vi "Write_From_Dash_Values_To_NT_Ready_Arrays.vi"(0 "Pages":refnum<vi>[](array[refnum])) -> (1 "Names":string[](array[string]), 2 "Values":string[](array[string]))   [LabVIEW 2019]
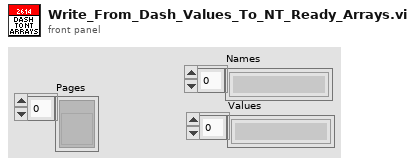
[diagram p1: front panel]
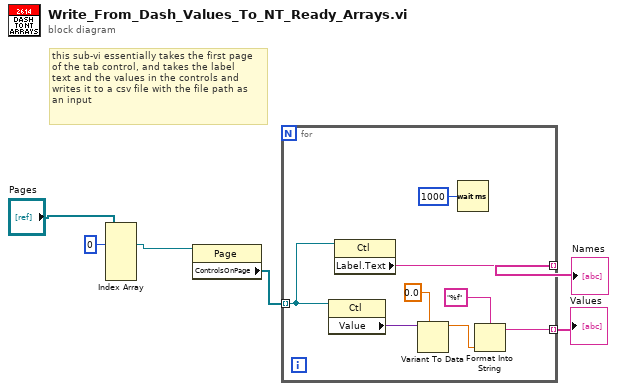
[diagram p0: block diagram]
diagram:
  # "this sub-vi essentially takes the first page\nof the tab control, and takes the label\ntext and the values in the controls and \nwrites it to a csv file with the file path as\nan input"
  n1 = Index Array(array="Pages", index #1=0 ("index")) -> (element #1=w6:refnum<vi>)  [unwired: 4 in, 4 out]
  n2 = property class="Page"(reference=w6) -> ("ControlsOnPage"=w3:refnum<vi>[])  [unwired: 1 in, 2 out]
  n3 = for {
    tunnel: w3 -> [w13] mode=indexing
    tunnel: [w14] -> w2 mode=indexing
    tunnel: [w7] -> w1 mode=indexing
    n4 = property class="Ctl"(reference=w13) -> ("Value"=w12:variant)  [unwired: 1 in, 2 out]
    n5 = property class="Ctl"(reference=w13) -> ("Label.Text"=w14:string)  [unwired: 1 in, 2 out]
    n6 = Variant To Data(type=0.0, Variant=w12) -> (data=w9:dbl)  [unwired: 1 in, 1 out]
    n7 = Wait (ms)(milliseconds to wait=u32 1000) -> ()  [unwired: 1 out]
    n8 = Format Into String(format string="%f", w9) -> (resulting string=w7:string)  [unwired: 2 in, 1 out]
  }
  "Names" <- w2
  "Values" <- w1
